vi "JPszczola_biletomat.vi"() -> ()   [LabVIEW 2020]
panel:
  in  "stop 2":bool
  in  "Enum":T1(ring)
  out "Wrzucono":dbl
  out "Razem":dbl
  out "Ilosc Ulg":dbl
  out "Ilosc norm":dbl
  in  "stop":bool
  out "Time Stamp":timestamp format="%<%X\n%x>T"
  in  "5 PLN":bool
  in  "2 PLN":bool
  in  "1 PLN":bool
  in  "50 gr":bool
  in  "20 gr":bool
  in  "10 gr":bool
  out "Boolean 3":bool
  in  "Rezygnuje":bool
  in  "Kupuje":bool
  in  "Remove  Ulg":bool
  in  "Add  Ulg":bool
  in  "Remove Norm":bool
  in  "Add Norm":bool
  out "Parameters":cluster{"Cena Norm":dbl, "Cena ulg":dbl}
  # "Biletomat"
  # "Razem"
  # "Wrzucono"
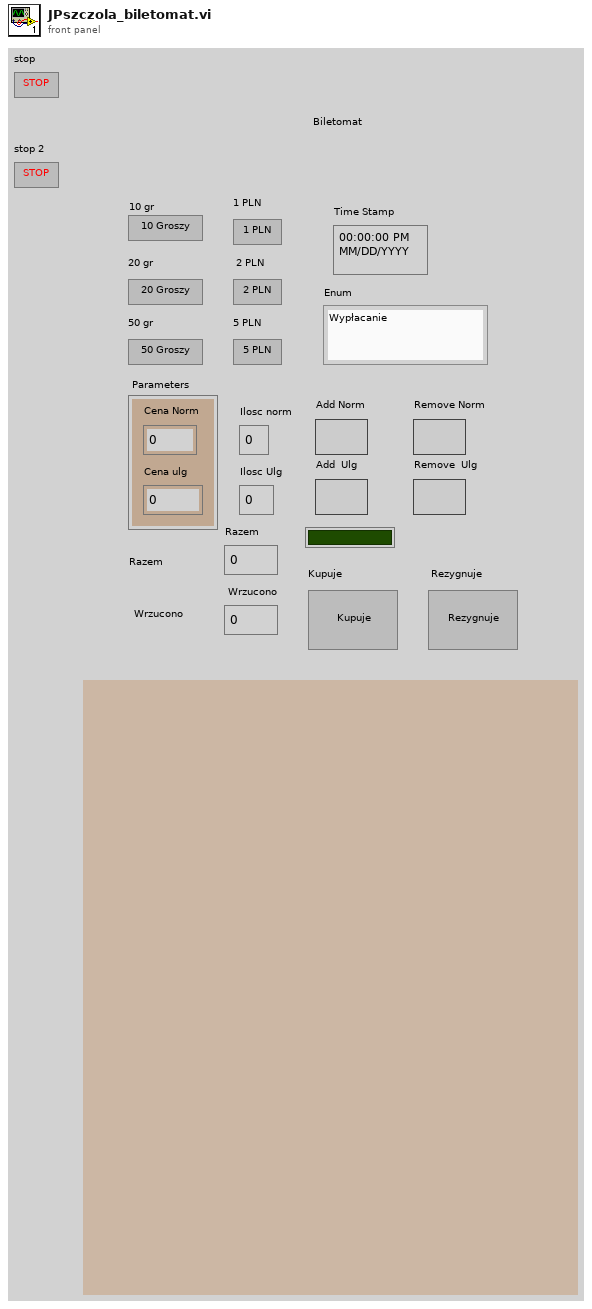
[diagram p1: front panel]
types:
  T1 = enum16{"Wypłacanie", "Wprowadź gotówke", "State1", "State2"}
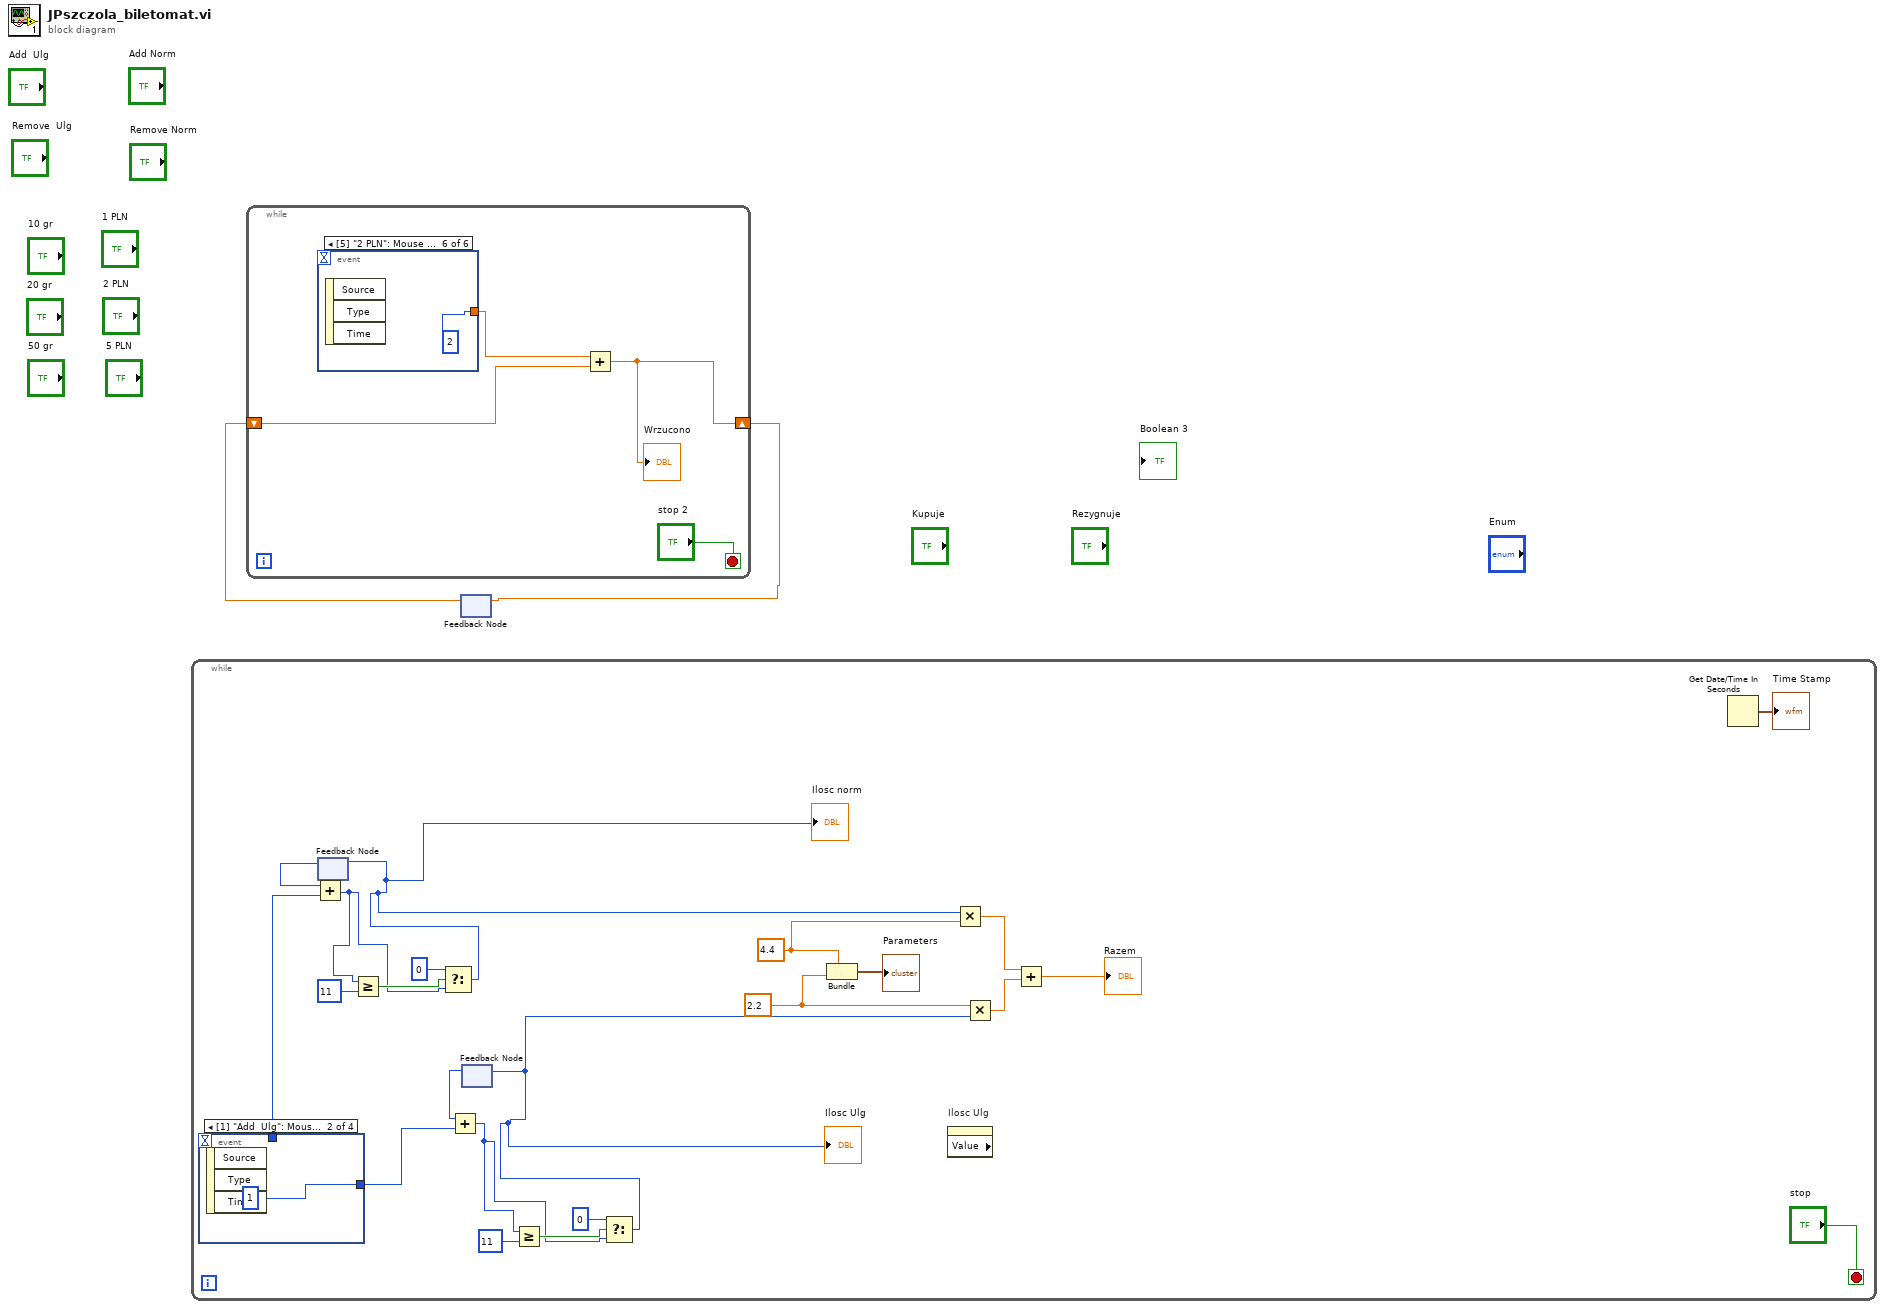
[diagram p0: block diagram]
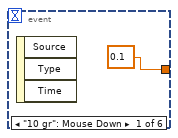
[diagram p2: hidden frame]
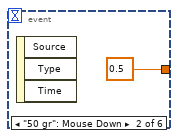
[diagram p3: hidden frame]
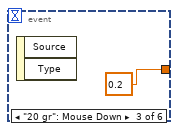
[diagram p4: hidden frame]
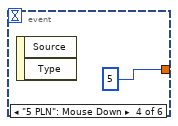
[diagram p5: hidden frame]
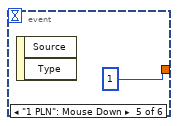
[diagram p6: hidden frame]
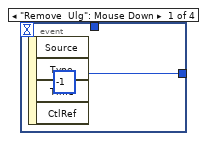
[diagram p7: hidden frame]
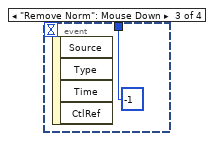
[diagram p8: hidden frame]
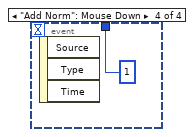
[diagram p9: hidden frame]
diagram:
  n1 = while {
    stop <- "stop" stop-if-true
    w18 = 2.2 ("Cena ulg")
    w17 = 4.4 ("Cena Norm")
    n2 = event shown="[1] \"Add  Ulg\": Mouse Down" {
      selector: _ -> [_ _ _ _]
      dyn-events: _ -> [_ _ _ _]
      timeout: _ -> [_ _ _ _]
      tunnel: [-1 1 _ _] -> w16
      tunnel: [_ _ -1 1] -> w14
      event "Remove  Ulg": Mouse Down {
        n3 = event-data() -> ()  [unwired: 1 in, 4 out]
      }
      event "Add  Ulg": Mouse Down {
        n4 = event-data() -> ()  [unwired: 1 in, 3 out]
      }
      event "Remove Norm": Mouse Down {
        n5 = event-data() -> ()  [unwired: 1 in, 4 out]
      }
      event "Add Norm": Mouse Down {
        n6 = event-data() -> ()  [unwired: 1 in, 3 out]
      }
    }
    n7 = feedback #1() -> (w15:i32)  [unwired: 1 in]
    n8 = Add(x=w15, y=w14) -> (x+y=w5:i32)
    n9 = Greater Or Equal?(x=w5, y=11) -> (x >= y?=w7:bool)
    n10 = Select(t=0, s=w7, f=w5) -> (s? t:f=w4:i32)
    "Ilosc norm" <- w4
    n11 = feedback-in #1(w4) -> ()
    n12 = feedback #2() -> (w3:i32)  [unwired: 1 in]
    n13 = Add(x=w3, y=w16) -> (x+y=w11:i32)
    n14 = Greater Or Equal?(x=w11, y=11) -> (x >= y?=w12:bool)
    n15 = Select(t=0, s=w12, f=w11) -> (s? t:f=w10:i32)
    "Ilosc Ulg" <- w10
    n16 = feedback-in #2(w10) -> ()
    n17 = Bundle("Cena Norm"=w17, "Cena ulg"=w18) -> (→"Parameters":cluster{"Cena Norm":dbl, "Cena ulg":dbl})  [unwired: 1 in]
    n18 = property on="Ilosc Ulg" class="DigNum (strict)" props=["Value"]() -> ()  [unwired: 2 in, 3 out]
    n19 = Multiply(x=w4, y=w17) -> (x*y=w22:dbl)
    n20 = Multiply(x=w18, y=w10) -> (x*y=w21:dbl)
    n21 = Add(x=w22, y=w21) -> (x+y=→"Razem":dbl)
    n22 = Get Date/Time In Seconds() -> (seconds since 1Jan1904=→"Time Stamp":timestamp)
  }
  n23 = feedback #3() -> (w2:dbl)  [unwired: 1 in]
  n24 = while {
    shift-right: [w29] -> w1
    shift-left: w2 -> [w32]
    stop <- "stop 2" stop-if-true
    n25 = event shown="[5] \"2 PLN\": Mouse Down" {
      selector: _ -> [_ _ _ _ _ _]
      dyn-events: _ -> [_ _ _ _ _ _]
      timeout: _ -> [_ _ _ _ _ _]
      tunnel: [0.1 0.5 0.2 5 1 2] -> w31
      event "10 gr": Mouse Down {
        n26 = event-data() -> ()  [unwired: 1 in, 3 out]
      }
      event "50 gr": Mouse Down {
        n27 = event-data() -> ()  [unwired: 1 in, 3 out]
      }
      event "20 gr": Mouse Down {
        n28 = event-data() -> ()  [unwired: 1 in, 2 out]
      }
      event "5 PLN": Mouse Down {
        n29 = event-data() -> ()  [unwired: 1 in, 2 out]
      }
      event "1 PLN": Mouse Down {
        n30 = event-data() -> ()  [unwired: 1 in, 2 out]
      }
      event "2 PLN": Mouse Down {
        n31 = event-data() -> ()  [unwired: 1 in, 3 out]
      }
    }
    n32 = Add(x=w31, y=w32) -> (x+y=w29:dbl)
    "Wrzucono" <- w29
  }
  n33 = feedback-in #3(w1) -> ()
